vi "global_variables.vi"() -> ()   [LabVIEW 2019]
panel:
  in  "Homing / Triggering lines 2":tag="DAQ2/port0/line17"
  in  "Homing / Triggering lines":tag="DAQ2/port0/line17"
  in  "PDU IP or Hostname":string="172.20.125.112"
  in  "Watchdog lines":tag="WDDAQ/port1/line0:3"
  in  "motor driver lines":tag="DAQ2/port0/line0:2"
  in  "Shift output channel 2":tag="DAQ2/ao3"
  in  "TX channel 2":tag="DAQ2/ao1"
  in  "LSB":dbl=8.0
  in  "Rotary encoder lines":tag="DAQ2/port0/line8:15"
  in  "Shift output channel 1":tag="DAQ2/ao2"
  in  "TX channel 1":tag="DAQ2/ao0"
  in  "Analog input start trigger":tag="/DAQ2/ai/StartTrigger"
  in  "Shift curr. meas. channel mode":i32(ring)=10106 items=["Default"=-1, "RSE"=10083, "NRSE"=10078, "Differential"=10106, "Pseudodifferential"=12529]
  in  "RX channel mode":i32(ring)=10083 items=["Default"=-1, "RSE"=10083, "NRSE"=10078, "Differential"=10106, "Pseudodifferential"=12529]
  in  "Shift current meas. channel":tag="DAQ2/ai2"
  in  "RX channel":tag="DAQ2/ai0"
  in  "Device Name":tag="DAQ2"
  in  "TX cycles":i32=150
  in  "Receive range":dbl=1.0
  in  "Receive frequency":dbl=75000.0 format="%#_6p"
  in  "sample rate digital out":dbl=40000.0 format="%#_6p"
  in  "Transmit amplitude":dbl=3.3
  in  "Transmit frequency":dbl=25000.0 format="%#_6p"
  in  "sample rate":dbl=500000.0 format="%#_6p"
  out "Master caution":bool
  out "Stop sub-vi":bool
  # "DAQ and transmit settings"
  # "Receive settings"
  # "DAQ channel selection for experiment"
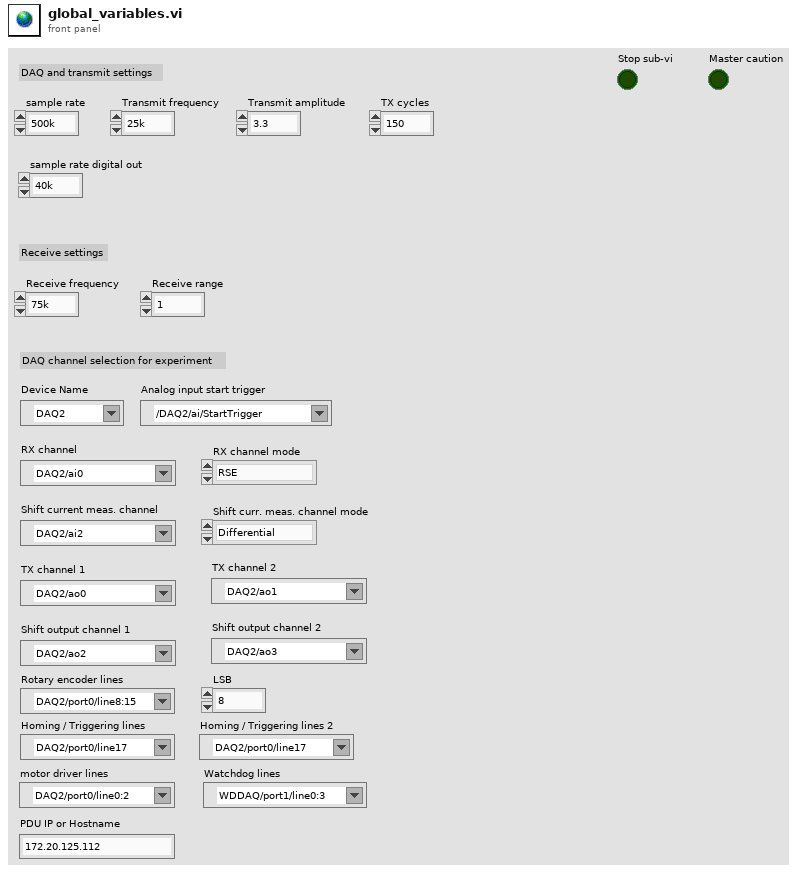
[diagram p1: front panel]
diagram:
